vi "Change ILC Mode.vi"(8 "error in (no error)":errorcluster, 10 "Mode":u16, 11 "Model in":refnum<class "Model.lvclass">) -> (0 "error out":errorcluster, 3 "Model out":refnum<class "Model.lvclass">)   [LabVIEW 2016, in "Model.lvclass"]
uses:
  Model.lvclass
  Model.lvclass/Model.ctl
  Common_RT_ILC/ILC/ILC.lvclass/ILC.ctl
  Common_RT_Modbus/DynamicFrameParser/DynamicFrameParser.lvclass
  Common_RT_FAILC/FAILC/FAILC.lvclass
  D:/Code/ts_FAMT/Common_RT_ILC/ILC/ILC.lvclass
  Modbus/DesktopModbus/DesktopModbus.lvclass
  Common_RT_ILC/ILC/ILC.lvclass
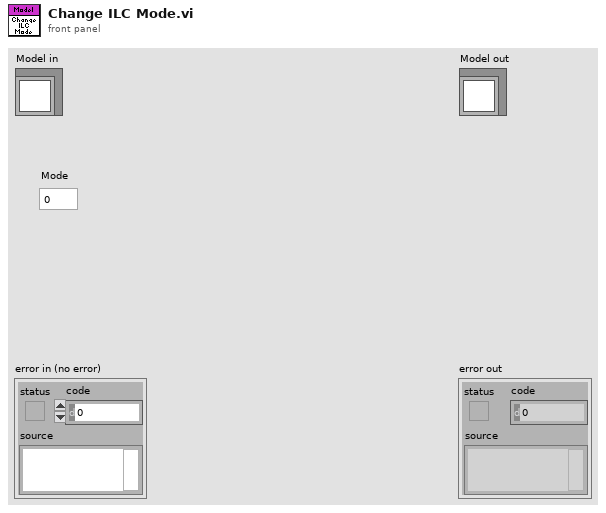
[diagram p1: front panel]
types:
  T1 = typedef "RTILC.lvlib/ILCData.ctl" = cluster{"Constants":T2, "Command":T3, "Telemetry":T5, "Responses":T6}
  T2 = typedef "RTILC.lvlib/ILCConstants.ctl" = cluster{"Subnet":u8, "Address":u8}
  T3 = typedef "RTILC.lvlib/ILCCommand.ctl" = cluster{"ILCMode":u16, "TemporaryAddress":u8, "ADCScanRate":T4, "ADCChannel":u8, "ADCOffset":sgl, "ADCSensitivity":sgl}
  T4 = typedef "RTILC.lvlib/ILCScanRates.ctl" = u8
  T5 = typedef "RTILC.lvlib/ILCTelemetry.ctl" = cluster{"UniqueID":u64, "FirmwareType":u8, "NetworkNodeType":u8, "ILCOption":u8, "NetworkNodeOption":u8, "MajorRevision":u8, "MinorRevision":u8, "FirmwareName":string, "ILCMode":u16, "MajorFault":bool, "MinorFault":bool, "FaultOverride":bool, "UniqueIDCRCMismatch":bool, "AppTypeNodeTypeMismatch":bool, "AppMissing":bool, "AppCRCMismatch":bool, "TEDSNotFound":bool, "TEDS1Mismatch":bool, "TEDS2Mismatch":bool, "WatchdogResetDetected":bool, "BrownoutDetected":bool, "EventTrapResetDetected":bool, "TemporaryAddress":u8, "ADCScanRate":T4, "DAC1":u16, "DAC2":u16, "DAC3":u16, "DAC4":u16, "MainADCCalibrationK":sgl[], "MainSensorOffset":sgl[], "MainSensorSensitivity":sgl[], "BackupADCCalibrationK":sgl[], "BackupSensorOffset":sgl[], "BackupSensorSensitivity":sgl[]}
  T6 = typedef "RTILC.lvlib/ILCResponses.ctl" = cluster{"ReportServerID":T7, "ReportServerStatus":T7, "ILCMode":T7, "SetTemporaryAddress":T7, "Reset":T7, "ADCScanRate":T7, "ADCOffsetSensitivity":T7, "ReadDAC":T7, "ReadCalibration":T7}
  T7 = typedef "RTModbus.lvlib/ExceptionCodes.ctl" = u16
  T8 = typedef "RTModbus.lvlib/Frame.ctl" = cluster{"Data":u8[], "WaitForTrigger":bool, "WaitForRx":u16, "TriggerIRQ":bool, "DelayTicks":u16, "DelayMicroseconds":u16, "DelayMilliseconds":u16}
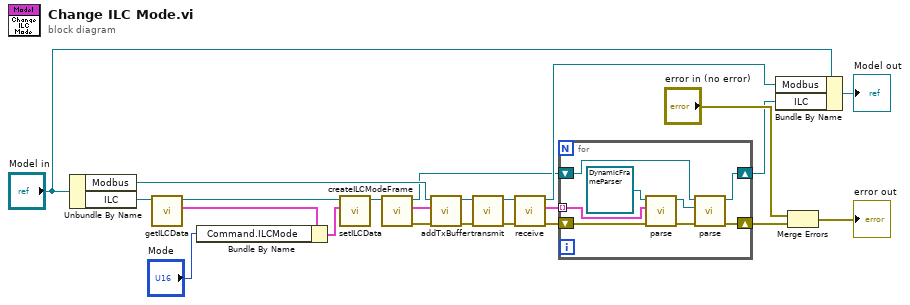
[diagram p0: block diagram]
diagram:
  n1 = Unbundle By Name("Model in") -> ("Modbus"=w16:refnum<class "DesktopModbus.lvclass">, "ILC"=w22:refnum<class "FAILC.lvclass">)
  n2 = call "getILCData.vi"("ILC in"=w22) -> ("ILCData"=w21:T1, "ILC out"=w18:refnum<class "FAILC.lvclass">)  [unwired: 9 in]
  n3 = Bundle By Name(cluster=w21, "Command.ILCMode"="Mode") -> (w19:T1)
  n4 = call "setILCData.vi"("ILCData"=w19, "ILC in"=w18) -> ("ILC out"=w17:refnum<class "FAILC.lvclass">)  [unwired: 9 in]
  n5 = call "createILCModeFrame.vi"("ILC in"=w17) -> ("error out"=w12:errorcluster, "Frame"=w15:T8, "ILC out"=w3:refnum<class "FAILC.lvclass">)  [unwired: 8 in]
  n6 = call-dynamic "addTxBuffer.vi"("error in (no error)"=w12, "Frame"=w15, "DesktopModbus in"=w16) -> ("error out"=w11:errorcluster, "DesktopModbus out"=w14:refnum<class "DesktopModbus.lvclass">)  [unwired: 7 in]
  n7 = call-dynamic "transmit.vi"("error in (no error)"=w11, "DesktopModbus in"=w14) -> ("error out"=w10:errorcluster, "DesktopModbus out"=w13:refnum<class "DesktopModbus.lvclass">)  [unwired: 8 in]
  n8 = call-dynamic "receive.vi"("error in (no error)"=w10, "DesktopModbus in"=w13) -> ("error out"=w4:errorcluster, "Data"=w5:T8[], "DesktopModbus out"=w7:refnum<class "DesktopModbus.lvclass">)  [unwired: 7 in]
  n9 = for {
    tunnel: w5 -> [w29] mode=indexing
    shift-right: [w26] -> w2
    shift-left: w4 -> [w28]
    shift-right: [w24] -> w1
    shift-left: w3 -> [w25]
    n10 = call "parse.vi"("error in (no error)"=w28, "Frame"=w29, "FrameParser in"=refnum<class "DynamicFrameParser.lvclass"> refnum ("RTModbus.lvlib:DynamicFrameParser.lvclass")) -> ("error out"=w27:errorcluster, "FrameParser out"=w31:refnum<class "DynamicFrameParser.lvclass">)  [unwired: 7 in]
    n11 = call-dynamic "parse.vi"("error in (no error)"=w27, "DynamicFrameParser"=w31, "FAILC in"=w25) -> ("error out"=w26:errorcluster, "FAILC out"=w24:refnum<class "FAILC.lvclass">)  [unwired: 6 in, 1 out]
  }
  n12 = Bundle By Name(cluster="Model in", "Modbus"=w7, "ILC"=w1) -> (→"Model out":refnum<class "Model.lvclass">)
  n13 = Merge Errors("error in (no error)", w2) -> (→"error out":errorcluster)
